vi "Add Or Replace String Array.vi"(8 "String":string="empty", 9 "Index":i32, 11 "Array In":string[](array[string])) -> (3 "Array Out":string[](array[string]))   [LabVIEW 2013]
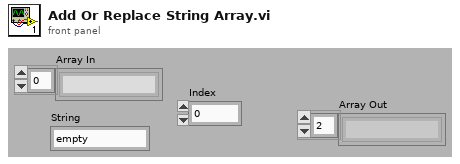
[diagram p1: front panel]
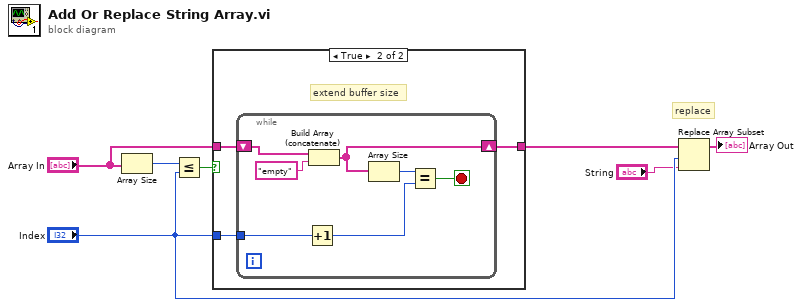
[diagram p0: block diagram]
diagram:
  # "replace"
  n1 = Array Size(array="Array In") -> (size(s)=w7:i32)
  n2 = Less Or Equal?(x=w7, y="Index") -> (x <= y?=w6:bool)
  n3 = case shown="True" w6 {
    tunnel: "Array In" -> [w8 w11]
    tunnel: [w8 w10] -> w5
    tunnel: "Index" -> [_ w9]
    frame False {
    }
    frame True {
      # "extend buffer size"
      n4 = while {
        shift-right: [w17] -> w10
        shift-left: w11 -> [w18]
        tunnel: w9 -> [w15]
        stop <- w14 stop-if-true
        n5 = Increment(x=w15) -> (x+1=w13:i32)
        n6 = Build Array (concatenate)(w18, "empty") -> (w17:string[])
        n7 = Array Size(array=w17) -> (size(s)=w16:i32)
        n8 = Equal?(x=w16, y=w13) -> (x = y?=w14:bool)
      }
    }
  }
  n9 = Replace Array Subset(array=w5, new element="String", index="Index") -> (→"Array Out":string[])
